vi "Thin Etalon Linewidth Sweep.vi"() -> ()   [LabVIEW 2013]
uses:
  Custom Controls/Thin Etalon Linewidth Sweep States.ctl
  <vilib>/Utility/error.llb/DialogType.ctl
panel:
  in  "Linewidth Threshold":dbl=7.0 format="%#_13g"
  out "Etalon Position History":i32[](graph)
  out "Task":T1
  out "WS7 Ch1 Linewidth":dbl format="%.2f"
  out "WS7 Ch1 Wavenumber":dbl format="%.4f"
  out "MPM Ch7 Reference Power":dbl format="%.3p"
  out "Thick Etalon Position":i32
  in  "Thin Etalon Position Setpoint":i32
  out "Thin Etalon Position":i32
  in  "Export Data":bool
  in  "Save to Image":bool
  out "XY Graph":cluster{cluster{"Int32":i32, "Double":dbl}[]}[](graph)
  in  "reset":bool
  out "Underexposed!":bool
  out "Time Elapsed":dbl
  in  "hysteresis correction":i32
  in  "sweep stepping speed (ms)":u32=25
  in  "Start Sweep":bool
  out "Done":bool
  out "Error Finding Center":bool
  out "right edge":i32
  out "left edge":i32
  out "Thin Etalon Position":i32(slide) scale=-5.0..15.0
  out "Center Position":i32
  in  "sweep steps":i32=5 min=1 max=50 step=1
  in  "stop":bool
  out "loop counter":i32
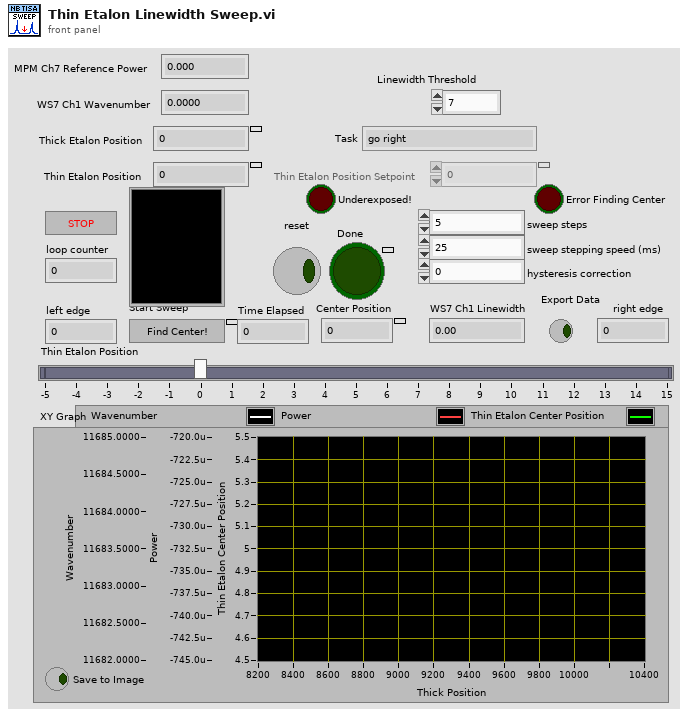
[diagram p1: front panel]
types:
  T1 = typedef "Thin Etalon Linewidth Sweep States.ctl" = enum16{"go right", "go left", "go more left", "go to center", "do nothing"}
  T2 = enum16{"open", "replace", "create", "open or create", "replace or create", "replace or create with confirmation"}
  T3 = typedef "imagedata.ctl" = cluster{"image type":i32, "image depth":i32, "image":u8[], "mask":u8[], "colors":u32[], "Rectangle":cluster{"left":i16, "top":i16, "right":i16, "bottom":i16}}
  T4 = typedef "DialogType.ctl" = u16
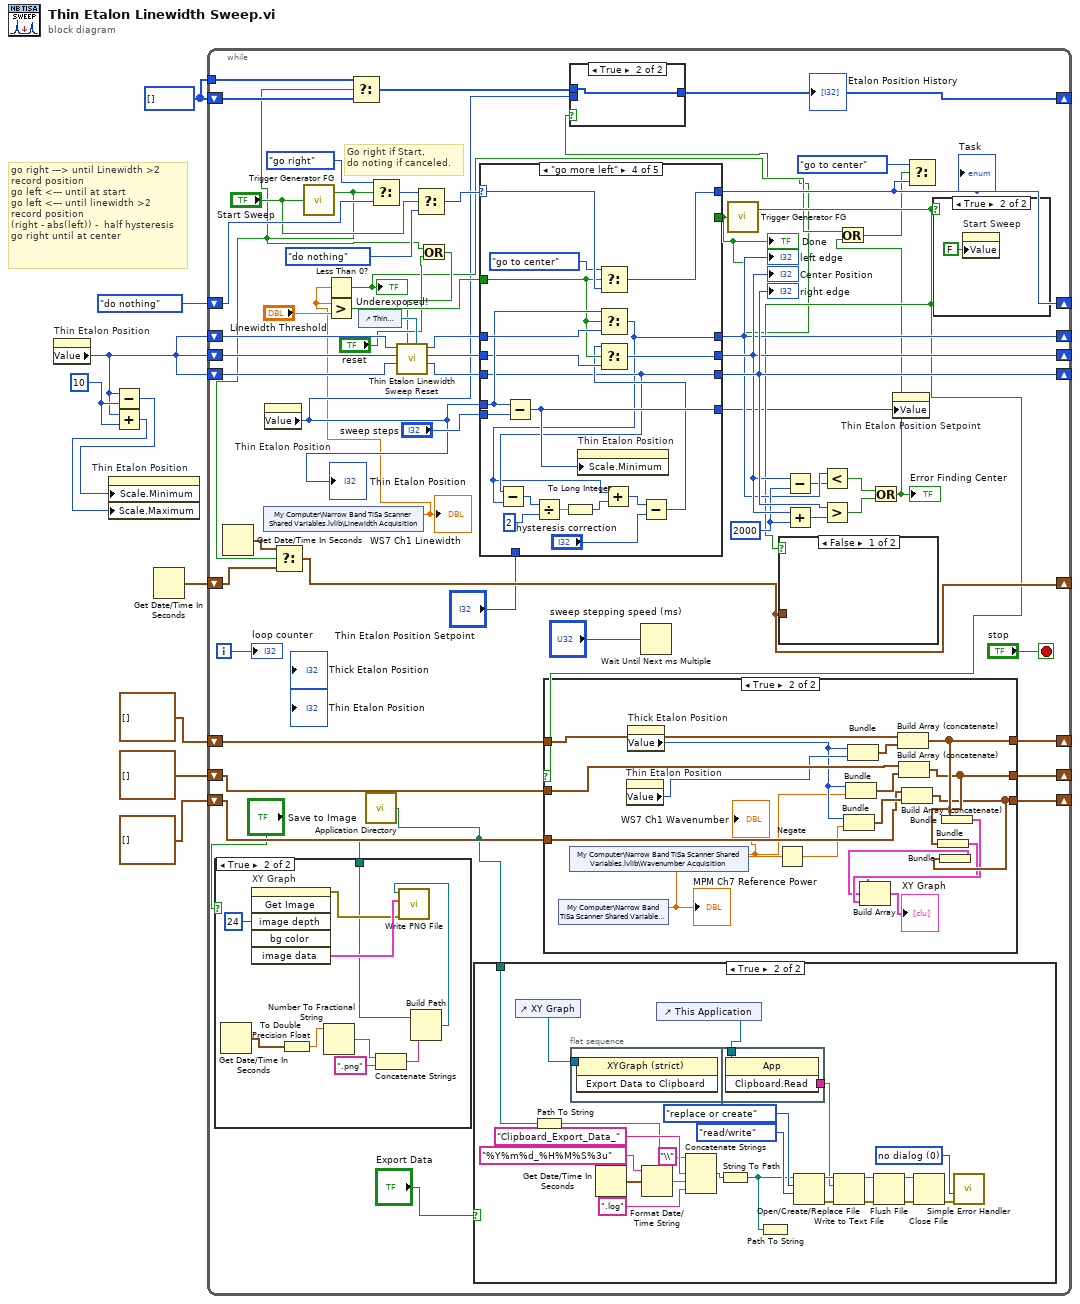
[diagram p0: block diagram]
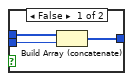
[diagram p2: hidden frame]
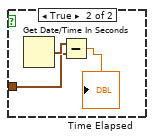
[diagram p6: hidden frame]
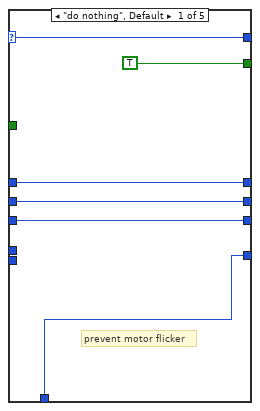
[diagram p8: hidden frame]
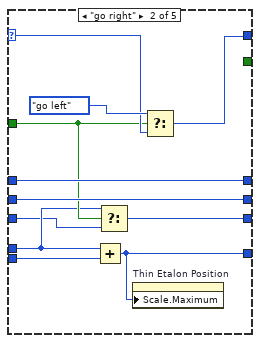
[diagram p9: hidden frame]
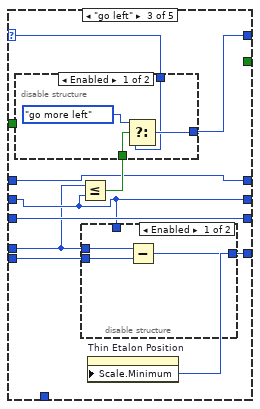
[diagram p10: hidden frame]
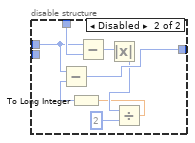
[diagram p11: hidden frame]
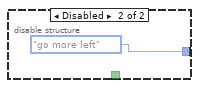
[diagram p12: hidden frame]
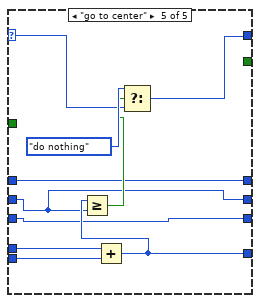
[diagram p13: hidden frame]
diagram:
  w1 = i32[] []
  w8 = 10
  # "go right ---> until Linewidth >2\nrecord position\ngo left <--- until at start\ngo left <--- until linewidth >2\nrecord position\n(right - abs(left)) -  half hysteresis\ngo right until at center"
  n1 = property on="Thin Etalon Position" class="DigNum (strict)"() -> ("Value"=w2:i32)  [unwired: 2 in, 2 out]
  n2 = Subtract(x=w2, y=w8) -> (x-y=w9:i32)
  n3 = Add(x=w2, y=w8) -> (x+y=w7:i32)
  n4 = property on="Thin Etalon Position" class="Slide (strict)"("Scale.Minimum"=w9, "Scale.Maximum"=w7) -> ()  [unwired: 2 in, 2 out]
  n5 = Get Date/Time In Seconds() -> (seconds since 1Jan1904=w6:timestamp)
  n6 = while {
    shift-right: [w51] -> _
    shift-left: Thin_Etalon_Linewidth_Sweep_States."do nothing" -> [w61]
    shift-right: [w56] -> _
    shift-left: w2 -> [w43]
    shift-right: [w58] -> _
    shift-left: w2 -> [w42]
    shift-right: [w60] -> _
    shift-left: w2 -> [w41]
    shift-right: [w48] -> _
    shift-left: w6 -> [w49]
    shift-right: [w36] -> _
    shift-left: cluster{"Int32":i32, "Int32":i32}[] [] -> [w35]
    shift-right: [w34] -> _
    shift-left: cluster{"Int32":i32, "Double":dbl}[] [] -> [w32]
    shift-right: [w33] -> _
    shift-left: cluster{"Int32":i32, "Double":dbl}[] [] -> [w31]
    shift-right: [w15] -> _
    shift-left: w1 -> [w18]
    tunnel: w1 -> [w19]
    i -> [w67]
    stop <- "stop" stop-if-true
    w57 = 2000
    # "Go right if Start,\ndo noting if canceled."
    n7 = Get Date/Time In Seconds() -> (seconds since 1Jan1904=w50:timestamp)
    n8 = shared-variable "My Computer\\Narrow Band TiSa Scanner Shared Variables.lvlib\\Linewidth Acquisition"() -> (w11:dbl)  [unwired: 1 in, 1 out]
    "WS7 Ch1 Linewidth" <- w11
    n9 = property on="Thin Etalon Position" class="DigNum (strict)"() -> ("Value"=w14:i32)  [unwired: 2 in, 2 out]
    "Thin Etalon Position" <- w14
    n10 = call "Trigger Generator FG.vi"("Boolean in"="Start Sweep") -> ("Rising Trigger out"=w16:bool)  [unwired: 1 out]
    n11 = Select(t=w50, s=w16, f=w49) -> (s? t:f=w48:timestamp)
    n12 = Less Than 0?(x=w11) -> (x < 0?=w21:bool)
    "Underexposed!" <- w21
    n13 = Greater?(x=w11, y="Linewidth Threshold") -> (0:w44:bool)
    n14 = Select(t=w19, s=w16, f=w18) -> (s? t:f=w17:i32[])
    n15 = control-ref of="Thin Etalon Position"() -> (w37:refnum<vi>)
    n16 = call <vilib>:"Application Directory.vi"() -> ("Application Directory"=w29:path)
    n17 = case shown="True" "Save to Image" {
      tunnel: w29 -> [_ w102]
      frame False {
      }
      frame True {
        n18 = Get Date/Time In Seconds() -> (seconds since 1Jan1904=w103:timestamp)
        n19 = invoke on="XY Graph" class="XYGraph (strict)" method="Get Image"("image depth"=24 ("Image Depth")) -> (error out=w105:errorcluster, "image data"=w106:T3)  [unwired: 5 in, 4 out]
        n20 = To Double Precision Float(number=w103) -> (double precision float=w104:dbl)
        n21 = Number To Fractional String(number=w104) -> (F-format string=w101:string)  [unwired: 3 in]
        n22 = Concatenate Strings(w101, ".png" ("string")) -> (w99:string)
        n23 = Build Path(base path=w102, name or relative path=w99) -> (appended path=w98:path)
        n24 = call <vilib>:"Write PNG File.vi"("error in (no error)"=w105, "image data"=w106, "path to PNG file"=w98) -> ()  [unwired: 7 in, 2 out]
      }
    }
    n25 = Select(t=Thin_Etalon_Linewidth_Sweep_States."go right", s=w16, f=w61) -> (s? t:f=w47:T1)
    n26 = Select(t=w47, s="Start Sweep", f=Thin_Etalon_Linewidth_Sweep_States."do nothing") -> (s? t:f=w46:T1)
    n27 = Or(x=w16, y="reset") -> (x .or. y?=w24:bool)
    n28 = call "Thin Etalon Linewidth Sweep Reset.vi"("slide reference"=w37, "reset"=w24, "Right in"=w41, "center in"=w42, "left in"=w43) -> ("Right out"=w38:i32, "center out"=w39:i32, "left out"=w40:i32)  [unwired: 4 in]
    n29 = case shown="True" "Export Data" {
      tunnel: w29 -> [_ w76]
      frame False {
      }
      frame True {
        w88 = T4 0 items=["no dialog", "OK message", "continue or stop message", "OK message + warnings", "continue/stop + warnings"] ("type of dialog (OK msg:1)")
        n30 = control-ref of="XY Graph"() -> (w75:refnum<vi>)
        n31 = Path To String(path=w76) -> (string=w73:string)
        n32 = flat-sequence {
          tunnel: w75 -> [w95]
          tunnel: [w97] -> w91
          tunnel: w74 -> [w96]
          frame #0 {
            n33 = invoke on="Invoke Node" class="XYGraph (strict)" method="Export Data to Clipboard"(reference=w95) -> ()  [unwired: 2 in, 3 out]
          }
          frame #1 {
            n34 = invoke class="App" method="Clipboard.Read"(reference=w96) -> ("Read Clipbrd"=w97:string)  [unwired: 2 in, 2 out]
          }
        }
        n35 = Get Date/Time In Seconds() -> (seconds since 1Jan1904=w94:timestamp)
        n36 = Format Date/Time String(time format string (%c)="%Y%m%d_%H%M%S%3u", seconds (now)=w94) -> (date/time string=w86:string)  [unwired: 1 out]
        n37 = control-ref of="This Application"() -> (w74:refnum<vi>)
        n38 = Concatenate Strings(w73, "\\" ("string"), "Clipboard_Export_Data_", w86, ".log" ("string")) -> (w90:string)
        n39 = String To Path(string=w90) -> (path=w78:path)
        n40 = Path To String(path=w78) -> ()  [unwired: 1 out]
        n41 = Open/Create/Replace File(file path (use dialog)=w78, operation (0:open)=T2."replace or create", access (0:read/write)=enum16{"read/write", "read-only", "write-only"}."read/write") -> (refnum out=w92:refnum<file>, error out=w93:errorcluster)  [unwired: 3 in, 1 out]
        n42 = Write to Text File(file (use dialog)=w92, text=w91, error in=w93) -> (refnum out=w83:refnum<file>, error out=w82:errorcluster)  [unwired: 1 in, 1 out]
        n43 = Flush File(refnum=w83, error in=w82) -> (refnum out=w84:refnum<file>, error out=w85:errorcluster)
        n44 = Close File(refnum=w84, error in=w85) -> (error out=w89:errorcluster)  [unwired: 1 out]
        n45 = call <vilib>:"Simple Error Handler.vi"("type of dialog (OK msg:1)"=w88, "error in (no error)"=w89) -> ()  [unwired: 3 in, 5 out]
      }
    }
    n46 = case shown="\"go more left\"" w46 {
      selector: w46 -> [w138 w146 w154 w192 w201]
      tunnel: w14 -> [_ w141 w150 w189 w199]
      tunnel: "sweep steps" -> [_ w149 w158 w188 w203]
      tunnel: [w133 w139 w151 w184 w196] -> w23
      tunnel: w44 -> [_ w142 _ w185 _]
      tunnel: [w138 w148 w157 w193 w200] -> w51
      tunnel: [w137 w145 w155 w177 w197] -> w56
      tunnel: w40 -> [w137 w145 w155 w190 w197]
      tunnel: [w136 w144 w152 w186 w195] -> w58
      tunnel: w39 -> [w136 w144 w152 w187 w195]
      tunnel: [w135 w143 w153 w181 w194] -> w60
      tunnel: w38 -> [w135 w140 w153 w181 w194]
      tunnel: [TRUE _ _ _ _] -> w12
      tunnel: "Thin Etalon Position Setpoint" -> [w133 _ _ _ _]
      frame "do nothing", Default {
        # "prevent motor flicker"
      }
      frame "go right" {
        n47 = Add(x=w141, y=w149) -> (x+y=w139:i32)
        n48 = Select(t=w141, s=w142, f=w140) -> (s? t:f=w143:i32)
        n49 = property on="Thin Etalon Position" class="Slide (strict)"("Scale.Maximum"=w139) -> ()  [unwired: 2 in, 2 out]
        n50 = Select(t=Thin_Etalon_Linewidth_Sweep_States."go left", s=w142, f=w146) -> (s? t:f=w148:T1)
      }
      frame "go left" {
        n51 = Less Or Equal?(x=w150, y=w152) -> (x <= y?=w156:bool)
        n52 = disable-structure shown="Enabled" {
          disable-tunnel: [w173 Thin_Etalon_Linewidth_Sweep_States."go more left"] -> w157
          disable-tunnel: w156 -> [w172 _]
          disable-tunnel: w154 -> [w171 _]
          frame Enabled {
            n53 = Select(t=Thin_Etalon_Linewidth_Sweep_States."go more left", s=w172, f=w171) -> (s? t:f=w173:T1)
          }
          frame Disabled {
          }
        }
        n54 = disable-structure shown="Enabled" {
          disable-tunnel: w158 -> [w161 _]
          disable-tunnel: w150 -> [w160 w167]
          disable-tunnel: [w159 w166] -> w151
          disable-tunnel: w152 -> [_ w169]
          frame Enabled {
            n55 = Subtract(x=w160, y=w161) -> (x-y=w159:i32)
          }
          frame Disabled {
            n56 = Subtract(x=w167, y=w169) -> (x-y=w168:i32)
            n57 = Absolute Value(x=w168) -> (abs(x)=w165:i32)
            n58 = Divide(x=w165, y=2) -> (x/y=w163:dbl)
            n59 = To Long Integer(number=w163) -> (32bit integer=w162:i32)
            n60 = Subtract(x=w167, y=w162) -> (x-y=w166:i32)
          }
        }
        n61 = property on="Thin Etalon Position" class="Slide (strict)"("Scale.Minimum"=w151) -> ()  [unwired: 2 in, 2 out]
      }
      frame "go more left" {
        n62 = Subtract(x=w189, y=w188) -> (x-y=w184:i32)
        n63 = property on="Thin Etalon Position" class="Slide (strict)"("Scale.Minimum"=w184) -> ()  [unwired: 2 in, 2 out]
        n64 = Select(t=Thin_Etalon_Linewidth_Sweep_States."go to center", s=w185, f=w192) -> (s? t:f=w193:T1)
        n65 = Select(t=w189, s=w185, f=w190) -> (s? t:f=w177:i32)
        n66 = Subtract(x=w181, y=w177) -> (x-y=w180:i32)
        n67 = Divide(x=w180, y=2) -> (x/y=w178:dbl)
        n68 = To Long Integer(number=w178) -> (32bit integer=w176:i32)
        n69 = Add(x=w177, y=w176) -> (x+y=w175:i32)
        n70 = Subtract(x=w175, y="hysteresis correction") -> (x-y=w183:i32)
        n71 = Select(t=w183, s=w185, f=w187) -> (s? t:f=w186:i32)
      }
      frame "go to center" {
        n72 = Add(x=w199, y=w203) -> (x+y=w196:i32)
        n73 = Greater Or Equal?(x=w196, y=w195) -> (x >= y?=w198:bool)
        n74 = Select(t=Thin_Etalon_Linewidth_Sweep_States."do nothing", s=w198, f=w201) -> (s? t:f=w200:T1)
      }
    }
    "Center Position" <- w58
    "right edge" <- w60
    "Done" <- w12
    "left edge" <- w56
    "Task" <- w51
    n75 = case shown="True" w12 {
      tunnel: w17 -> [w70 w71]
      tunnel: [w69 w71] -> w15
      tunnel: w14 -> [w68 _]
      frame False {
        n76 = Build Array (concatenate)(w70, w68) -> (w69:i32[])
      }
      frame True {
      }
    }
    "Etalon Position History" <- w15
    n77 = Wait Until Next ms Multiple(millisecond multiple="sweep stepping speed (ms)") -> ()  [unwired: 1 out]
    n78 = call "Trigger Generator FG.vi"("Boolean in"=w12) -> ("Rising Trigger out"=w27:bool)  [unwired: 1 out]
    n79 = case shown="True" w27 {
      tunnel: [w110 w122] -> w36
      tunnel: w35 -> [w110 w127]
      tunnel: [w109 w121] -> w34
      tunnel: [w108 w120] -> w33
      tunnel: w32 -> [w109 w124]
      tunnel: w31 -> [w108 w123]
      frame False {
      }
      frame True {
        n80 = shared-variable "My Computer\\Narrow Band TiSa Scanner Shared Variables.lvlib\\Power MPM"() -> (w112:dbl)  [unwired: 1 in, 1 out]
        "MPM Ch7 Reference Power" <- w112
        n81 = shared-variable "My Computer\\Narrow Band TiSa Scanner Shared Variables.lvlib\\Wavenumber Acquisition"() -> (w111:dbl)  [unwired: 1 in, 1 out]
        "WS7 Ch1 Wavenumber" <- w111
        n82 = property on="Thin Etalon Position" class="DigNum (strict)"() -> ("Value"=w114:i32)  [unwired: 2 in, 2 out]
        n83 = property on="Thick Etalon Position" class="DigNum (strict)"() -> ("Value"=w113:i32)  [unwired: 2 in, 2 out]
        n84 = Negate(x=w112) -> (-x=w115:dbl)
        n85 = Bundle("Value"=w113, w115) -> (w125:cluster{"Value":i32, dbl})  [unwired: 1 in]
        n86 = Bundle("Value"=w113, "Double"=w111) -> (w126:cluster{"Value":i32, "Double":dbl})  [unwired: 1 in]
        n87 = Bundle("Value"=w113, "Value"=w114) -> (w128:cluster{"Value":i32, "Value":i32})  [unwired: 1 in]
        n88 = Build Array (concatenate)(w127, w128) -> (w122:cluster{"Value":i32, "Value":i32}[])
        n89 = Build Array (concatenate)(w124, w126) -> (w121:cluster{"Value":i32, "Double":dbl}[])
        n90 = Build Array (concatenate)(w123, w125) -> (w120:cluster{"Value":i32, "Double":dbl}[])
        n91 = Bundle(w121) -> (w117:cluster{cluster{"Value":i32, "Double":dbl}[]})  [unwired: 1 in]
        n92 = Bundle(w120) -> (w116:cluster{cluster{"Value":i32, "Double":dbl}[]})  [unwired: 1 in]
        n93 = Bundle(w122) -> (w118:cluster{cluster{"Value":i32, "Value":i32}[]})  [unwired: 1 in]
        n94 = Build Array(w117, w116, w118) -> (→"XY Graph":cluster{cluster{"Value":i32, "Double":dbl}[]}[])
      }
    }
    n95 = case shown="False" w27 {
      tunnel: w48 -> [_ w130]
      frame False {
      }
      frame True {
        n96 = Get Date/Time In Seconds() -> (seconds since 1Jan1904=w131:timestamp)
        n97 = Subtract(x=w131, y=w130) -> (x-y=→"Time Elapsed":dbl)
      }
    }
    n98 = Subtract(x=w58, y=w57) -> (x-y=w55:i32)
    n99 = Add(x=w58, y=w57) -> (x+y=w59:i32)
    n100 = Less?(x=w56, y=w55) -> (x < y?=w54:bool)
    n101 = Greater?(x=w60, y=w59) -> (0:w53:bool)
    n102 = Or(x=w54, y=w53) -> (x .or. y?=w22:bool)
    "Error Finding Center" <- w22
    n103 = Or(x=w21, y=w22) -> (x .or. y?=w20:bool)
    n104 = property on="Thin Etalon Position Setpoint" class="DigNum (strict)"("Value"=w23) -> ()  [unwired: 2 in, 2 out]
    n105 = Select(t=Thin_Etalon_Linewidth_Sweep_States."go to center", s=w20, f=w51) -> ()  [unwired: 1 out]
    n106 = case shown="True" w27 {
      frame False {
      }
      frame True {
        n107 = property on="Start Sweep" class="Bool (strict)"("Value"=FALSE ("Start Sweep")) -> ()  [unwired: 2 in, 2 out]
      }
    }
    "loop counter" <- w67
  }
